vi "goal_with_force_array_Msg.vi"(8 "error in (no error)":errorcluster caption="错误输入（无错误）", 10 "值(信号)":T1(array[cluster]), 11 "GlobalPlannerPyPl输入":refnum<class "GlobalPlannerPyPl.lvclass">) -> (0 "error out":errorcluster caption="错误输出", 3 "GlobalPlannerPyPl输出":refnum<class "GlobalPlannerPyPl.lvclass">)   [LabVIEW 2014, in "GlobalPlannerPyPl.lvlib" / "GlobalPlannerPyPl.lvclass"]
uses:
  GlobalPlannerPyPl.lvclass
  GlobalPlannerPyPl.lvclass/GlobalPlannerPyPl.ctl
  Global_var/Global_var.vi
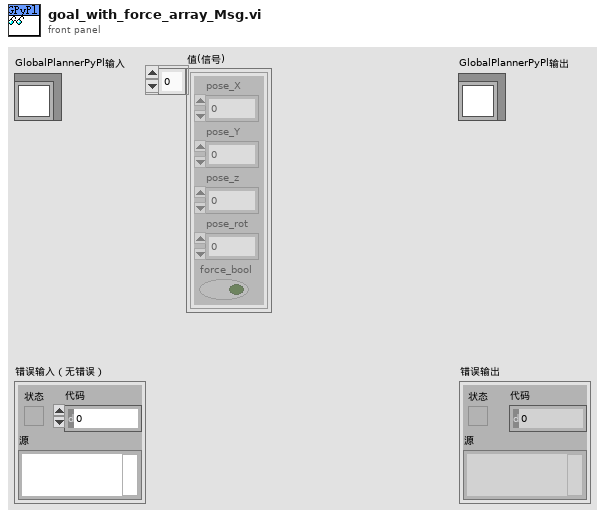
[diagram p1: front panel]
types:
  T1 = cluster{"pose_X":dbl, "pose_Y":dbl, "pose_z":dbl, "pose_rot":dbl, "force_bool":bool}[]
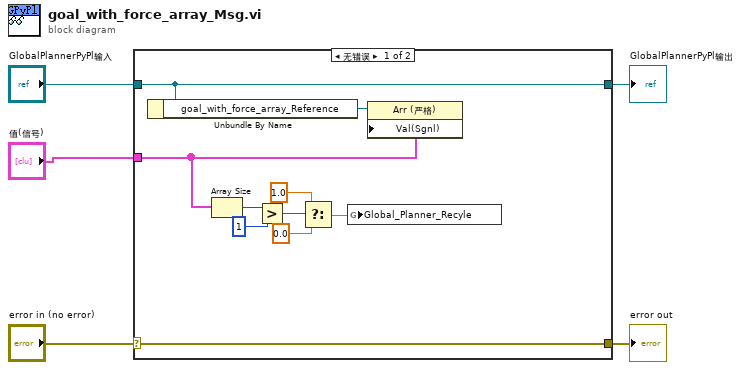
[diagram p0: block diagram]
diagram:
  n1 = case shown="无错误" "error in (no error)" {
    selector: "error in (no error)" -> [w15 w16]
    tunnel: [w15 w16] -> w4
    tunnel: [w14 w17] -> w2
    tunnel: "GlobalPlannerPyPl输入" -> [w14 w17]
    tunnel: "值(信号)" -> [w12 _]
    frame No Error {
      n2 = Unbundle By Name(w14) -> ("goal_with_force_array_Reference"=w13:refnum<vi>)
      n3 = Array Size(array=w12) -> (size(s)=w11:i32)
      n4 = Greater?(x=w11, y=1) -> (0:w9:bool)
      n5 = Select(t=1.0, s=w9, f=0.0) -> (s? t:f=w8:dbl)
      n6 = global write "Global_var.vi" "Global_Planner_Recyle"(w8) -> ()
      n7 = property class="Arr (严格)"(reference=w13, "Val(Sgnl)"=w12) -> ()  [unwired: 1 in, 2 out]
    }
    frame Error {
    }
  }
  "error out" <- w4
  "GlobalPlannerPyPl输出" <- w2
